vi "ExSetup1strip.vi"() -> ()   [LabVIEW 2010]
uses:
  Open-Close Hardware/CamHandle.vi
panel:
  out "ADC Speed":u32
  out "error out":errorcluster
  in  "error in (no error)":errorcluster
  in  "Timing Mode":u32(ring)=1 items=["N/A", "Timed Mode/Free run", "Trigger First (only PM)", "Strobed/Ext Sync", "Bulb Mode (PM only)", "Variable Timed mode (PM only)", "Flash Mode (only some PM)"]
  in  "x1":u32=1
  in  "x2":u32=1340
  in  "y1":u32=50
  in  "y2":u32=50
  in  "x bin":u32=1
  in  "y bin":u32=1
  in  "min block":u32=2
  in  "Num Min Block":u32=5
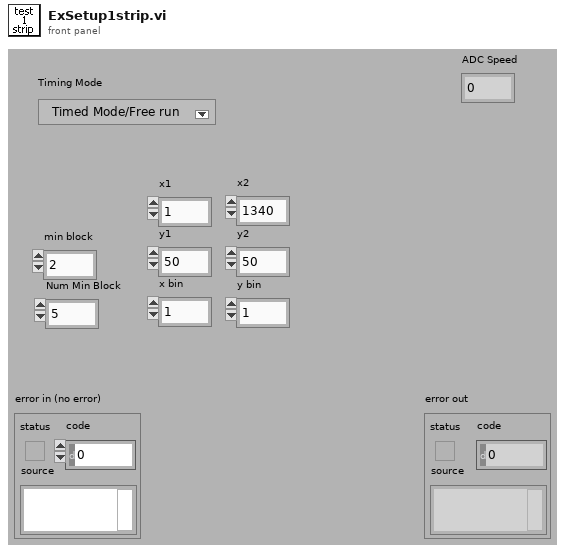
[diagram p1: front panel]
types:
  T1 = cluster{"x1":u32, "x2":u32, "x bin":u32, "y1":u32, "y2":u32, "y bin":u32}
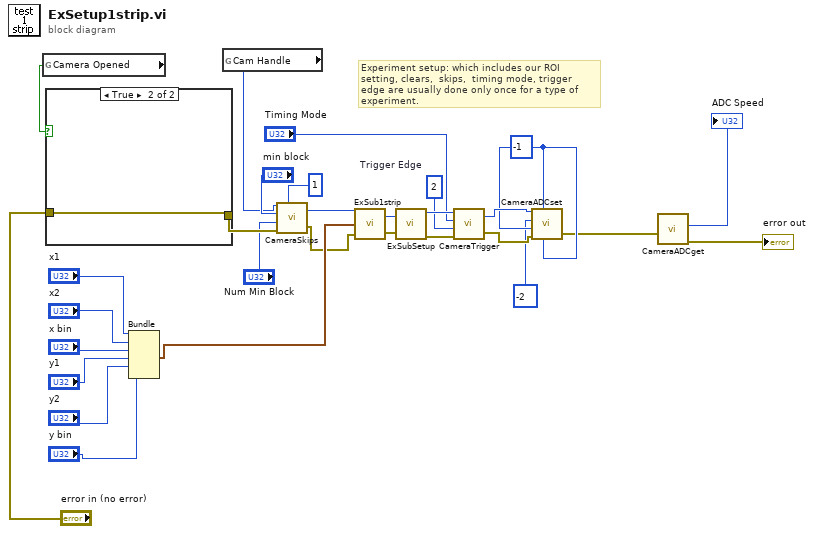
[diagram p0: block diagram]
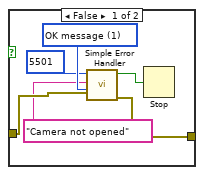
[diagram p2: hidden frame]
diagram:
  w23 = -1
  w27 = u32 2  # Trigger Edge
  # "Experiment setup: which includes our ROI setting, clears,  skips,  timing mode, trigger edge are usually done only once for a type of experiment."
  n1 = global read "CamHandle.vi" "Camera Opened"() -> (w26:bool)
  n2 = case shown="True" w26 {
    tunnel: "error in (no error)" -> [w34 w36]
    tunnel: [w33 w36] -> w13
    frame False {
      w35 = u16 1 items=["no dialog", "OK message", "continue or stop message"] ("type of dialog (OK msg:1)")
      n3 = call <vilib>:"Simple Error Handler.vi"("error code (no error:0)"=5501, "error source (\" \")"="Camera not opened", "type of dialog (OK msg:1)"=w35, "error in (no error)"=w34) -> ("error?"=w31:bool, "error out"=w33:errorcluster)  [unwired: 1 in, 3 out]
      n4 = Stop(stop? (T)=w31) -> ()
    }
    frame True {
    }
  }
  n5 = Bundle("x1"="x1", "x2"="x2", "x bin"="x bin", "y1"="y1", "y2"="y2", "y bin"="y bin") -> (w14:T1)  [unwired: 1 in]
  n6 = global read "CamHandle.vi" "Cam Handle"() -> (w6:u32)
  n7 = call <userlib>:"CameraSkips.vi"("Camera Handle"=w6, "Minimum Block Size"="min block", "Number of Minimum blocks"="Num Min Block", "error in"=w13, "Type of Skips"=1) -> ("Camera Handle"=w11:u32, "error out"=w12:errorcluster)
  n8 = call "ExSub1strip.vi"("error in (no error)"=w12, "strip 1"=w14, "Camera Handle"=w11) -> ("error out"=w21:errorcluster, "Camera Handle"=w7:u32)
  n9 = call "ExSubSetup.vi"("error in (no error)"=w21, "Camera Handle"=w7) -> ("error out"=w28:errorcluster, "Camera Handle"=w29:u32)
  n10 = call <userlib>:"CameraTrigger.vi"("error in"=w28, "Trigger Edge"=w27, "Timing Mode"="Timing Mode", "Camera Handle"=w29) -> ("error out"=w25:errorcluster, "Camera Handle"=w24:u32)
  n11 = call <userlib>:"CameraADCset.vi"("ADC offset"=w23, "Read Out port"=w23, "error in (no error)"=w25, "ADC Gain"=w23, "ADC Speed"=-2, "Camera Handle"=w24) -> ("error out"=w3:errorcluster)  [unwired: 1 out]
  n12 = call <userlib>:"CameraADCget.vi"("error in (no error)"=w3) -> ("ADC Speed"=→"ADC Speed":i32, "error out"=→"error out":errorcluster)  [unwired: 1 in, 6 out]
